vi "Find Nearest Lidar Point per Column.vi"(11 "Lidar Points":cluster{"X":dbl, "Y":dbl}[](array[cluster])) -> (3 "Nearest Point per Column":dbl[](array[numeric]))   [LabVIEW 2017]
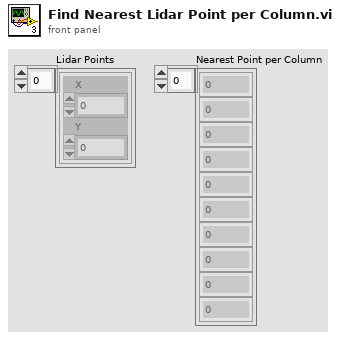
[diagram p1: front panel]
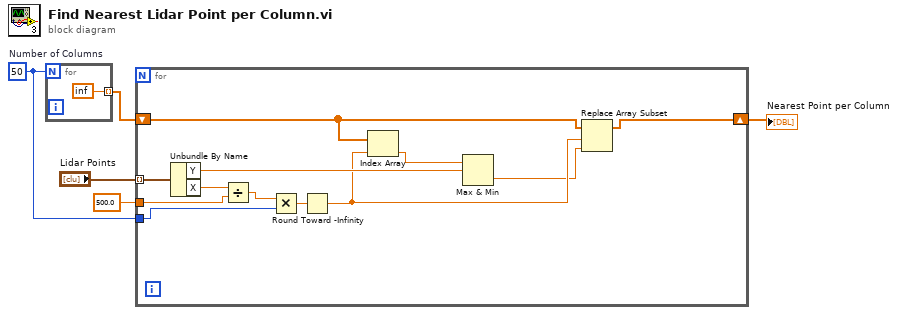
[diagram p0: block diagram]
diagram:
  w3 = 50  # Number of Columns
  n1 = for {
    N: w3 -> [_]
    tunnel: [inf] -> w4 mode=indexing
  }
  n2 = for {
    tunnel: "Lidar Points" -> [w18] mode=indexing
    shift-right: [w7] -> w1
    shift-left: w4 -> [w10]
    tunnel: w3 -> [w16]
    tunnel: 500.0 ("y") -> [w14]
    n3 = Unbundle By Name(w18) -> ("Y"=w11:dbl, "X"=w15:dbl)
    n4 = Divide(x=w15, y=w14) -> (x/y=w13:dbl)
    n5 = Multiply(x=w13, y=w16) -> (x*y=w17:dbl)
    n6 = Round Toward -Infinity(1:w17) -> (0:w9:dbl)
    n7 = Index Array(array=w10, index=w9) -> (element=w12:dbl)
    n8 = Max & Min(x=w12, y=w11) -> (min(x,y)=w8:dbl)  [unwired: 1 out]
    n9 = Replace Array Subset(array=w10, new element=w8, index=w9) -> (w7:dbl[])
  }
  "Nearest Point per Column" <- w1
